vi "Two Ball Not Working.vi"() -> ()   [LabVIEW 2013]
uses:
  Team Code/Robot Global Data.vi
panel:
  in  "Roller/Drive Ratio":dbl format="%#_13g"
  in  "Min. Power":dbl=0.25
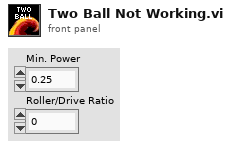
[diagram p1: front panel]
types:
  T1 = cluster{"FIRE!!!":bool, "Loader":bool, "Lock":bool, "Load":bool, "Pass":bool, "Grab":bool, "PANIC":bool, "Don't Cock":bool}
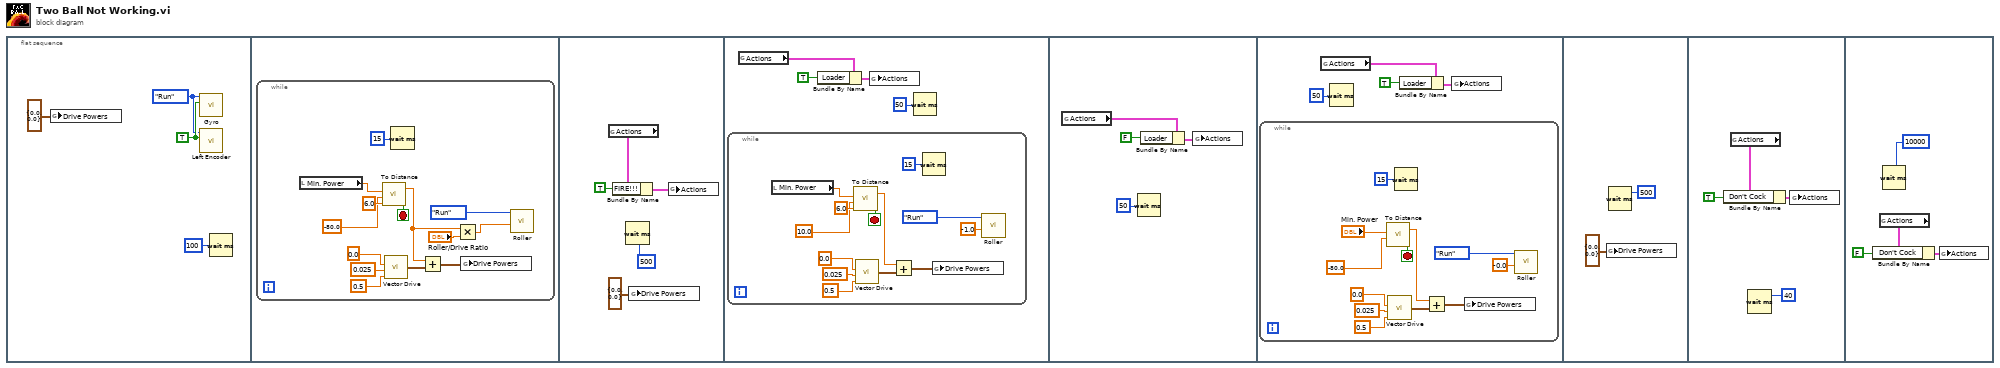
[diagram p0: block diagram]
diagram:
  n1 = flat-sequence {
    frame #0 {
      w3 = enum16{"Start", "Run", "End"}."Run" ("Enum")
      w4 = TRUE ("Reset")
      n2 = global write "Robot Global Data.vi" "Drive Powers"(cluster{"Right":dbl, "Left":dbl} {"Right"=0.0, "Left"=0.0} ("Drive Powers")) -> ()
      n3 = call "Gyro.vi"("Reset"=w4, "Enum"=w3) -> ()  [unwired: 9 in, 1 out]
      n4 = call "Left Encoder.vi"("Reset"=w4, "Enum"=w3) -> ()  [unwired: 8 in, 2 out]
      n5 = Wait (ms)(milliseconds to wait=u32 100) -> ()  [unwired: 1 out]
    }
    frame #1 {
      n6 = while {
        stop <- w18 stop-if-true
        n7 = local read "Min. Power"() -> (w7:dbl)
        n8 = call "To Distance.vi"("Tolerance"=6.0, "Destination Dist (in)"=-80.0 ("x"), "Min. Power"=w7) -> ("Reached Distance"=w18:bool, "Base Speed"=w10:dbl)  [unwired: 1 in]
        n9 = call "Vector Drive.vi"("Tolerance"=0.5, "Min. Power"=0.025, "Angle"=0.0) -> ("Motor Powers"=w14:cluster{"RMotor":dbl, "LMotor":dbl})  [unwired: 1 in]
        n10 = Wait (ms)(milliseconds to wait=u32 15) -> ()  [unwired: 1 out]
        n11 = Add(x=w10, y=w14) -> (x+y=w13:cluster{"RMotor":dbl, "LMotor":dbl})
        n12 = Multiply(x=w10, y="Roller/Drive Ratio") -> (x*y=w9:dbl)
        n13 = global write "Robot Global Data.vi" "Drive Powers"(w13) -> ()
        n14 = call "Roller.vi"("Power"=w9, "Enum"=enum16{"Start", "Run", "End"}."Run") -> ()  [unwired: 2 in]
      }
    }
    frame #2 {
      n15 = global read "Robot Global Data.vi" "Actions"() -> (w22:T1)
      n16 = Bundle By Name(cluster=w22, "FIRE!!!"=TRUE ("Primary Action")) -> (w23:T1)
      n17 = Wait (ms)(milliseconds to wait=u32 500) -> ()  [unwired: 1 out]
      n18 = global write "Robot Global Data.vi" "Drive Powers"(cluster{"Right":dbl, "Left":dbl} {"Right"=0.0, "Left"=0.0} ("Drive Powers")) -> ()
      n19 = global write "Robot Global Data.vi" "Actions"(w23) -> ()
    }
    frame #3 {
      n20 = while {
        stop <- w40 stop-if-true
        n21 = local read "Min. Power"() -> (w31:dbl)
        n22 = call "To Distance.vi"("Tolerance"=6.0, "Destination Dist (in)"=10.0 ("x"), "Min. Power"=w31) -> ("Reached Distance"=w40:bool, "Base Speed"=w32:dbl)  [unwired: 1 in]
        n23 = call "Vector Drive.vi"("Tolerance"=0.5, "Min. Power"=0.025, "Angle"=0.0) -> ("Motor Powers"=w36:cluster{"RMotor":dbl, "LMotor":dbl})  [unwired: 1 in]
        n24 = Add(x=w32, y=w36) -> (x+y=w35:cluster{"RMotor":dbl, "LMotor":dbl})
        n25 = Wait (ms)(milliseconds to wait=u32 15) -> ()  [unwired: 1 out]
        n26 = global write "Robot Global Data.vi" "Drive Powers"(w35) -> ()
        n27 = call "Roller.vi"("Power"=-1.0, "Enum"=enum16{"Start", "Run", "End"}."Run") -> ()  [unwired: 2 in]
      }
      n28 = global read "Robot Global Data.vi" "Actions"() -> (w26:T1)
      n29 = Bundle By Name(cluster=w26, "Loader"=TRUE ("Primary Action")) -> (w27:T1)
      n30 = global write "Robot Global Data.vi" "Actions"(w27) -> ()
      n31 = Wait (ms)(milliseconds to wait=u32 50) -> ()  [unwired: 1 out]
    }
    frame #4 {
      n32 = global read "Robot Global Data.vi" "Actions"() -> (w43:T1)
      n33 = Wait (ms)(milliseconds to wait=u32 50) -> ()  [unwired: 1 out]
      n34 = Bundle By Name(cluster=w43, "Loader"=FALSE ("Primary Action")) -> (w44:T1)
      n35 = global write "Robot Global Data.vi" "Actions"(w44) -> ()
    }
    frame #5 {
      n36 = while {
        stop <- w60 stop-if-true
        n37 = call "To Distance.vi"("Destination Dist (in)"=-80.0 ("x"), "Min. Power"="Min. Power") -> ("Reached Distance"=w60:bool, "Base Speed"=w53:dbl)  [unwired: 2 in]
        n38 = call "Vector Drive.vi"("Tolerance"=0.5, "Min. Power"=0.025, "Angle"=0.0) -> ("Motor Powers"=w56:cluster{"RMotor":dbl, "LMotor":dbl})  [unwired: 1 in]
        n39 = Wait (ms)(milliseconds to wait=u32 15) -> ()  [unwired: 1 out]
        n40 = Add(x=w53, y=w56) -> (x+y=w55:cluster{"RMotor":dbl, "LMotor":dbl})
        n41 = global write "Robot Global Data.vi" "Drive Powers"(w55) -> ()
        n42 = call "Roller.vi"("Power"=-0.0, "Enum"=enum16{"Start", "Run", "End"}."Run") -> ()  [unwired: 2 in]
      }
      n43 = global read "Robot Global Data.vi" "Actions"() -> (w47:T1)
      n44 = Wait (ms)(milliseconds to wait=u32 50) -> ()  [unwired: 1 out]
      n45 = Bundle By Name(cluster=w47, "Loader"=TRUE ("Primary Action")) -> (w46:T1)
      n46 = global write "Robot Global Data.vi" "Actions"(w46) -> ()
    }
    frame #6 {
      n47 = global write "Robot Global Data.vi" "Drive Powers"(cluster{"Right":dbl, "Left":dbl} {"Right"=0.0, "Left"=0.0} ("Drive Powers")) -> ()
      n48 = Wait (ms)(milliseconds to wait=u32 500) -> ()  [unwired: 1 out]
    }
    frame #7 {
      n49 = global read "Robot Global Data.vi" "Actions"() -> (w66:T1)
      n50 = Bundle By Name(cluster=w66, "Don't Cock"=TRUE ("Primary Action")) -> (w65:T1)
      n51 = Wait (ms)(milliseconds to wait=u32 40) -> ()  [unwired: 1 out]
      n52 = global write "Robot Global Data.vi" "Actions"(w65) -> ()
    }
    frame #8 {
      n53 = global read "Robot Global Data.vi" "Actions"() -> (w67:T1)
      n54 = Bundle By Name(cluster=w67, "Don't Cock"=FALSE ("Primary Action")) -> (w68:T1)
      n55 = Wait (ms)(milliseconds to wait=u32 10000) -> ()  [unwired: 1 out]
      n56 = global write "Robot Global Data.vi" "Actions"(w68) -> ()
    }
  }
